vi "Termék megnyitás.vi"(8 "error in":errorcluster) -> (0 "error out":errorcluster, 2 "File name":string, 3 "Termék cluster array":T1[](array[typedef]))   [LabVIEW 2014]
panel:
  out "text":string
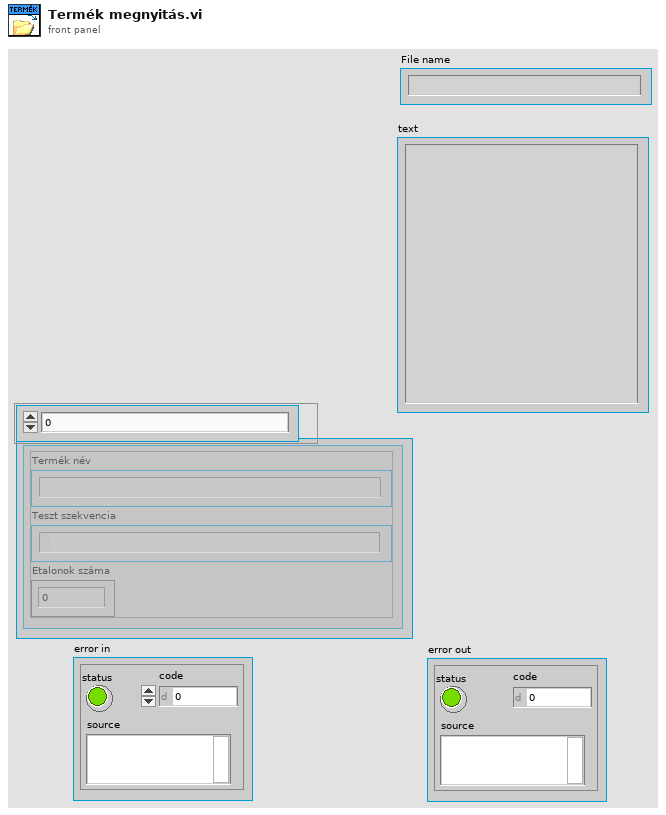
[diagram p1: front panel]
types:
  T1 = typedef "Termék cluster.ctl" = cluster{"Termék név":string, "Teszt szekvencia":path, "Etalonok száma":i8}
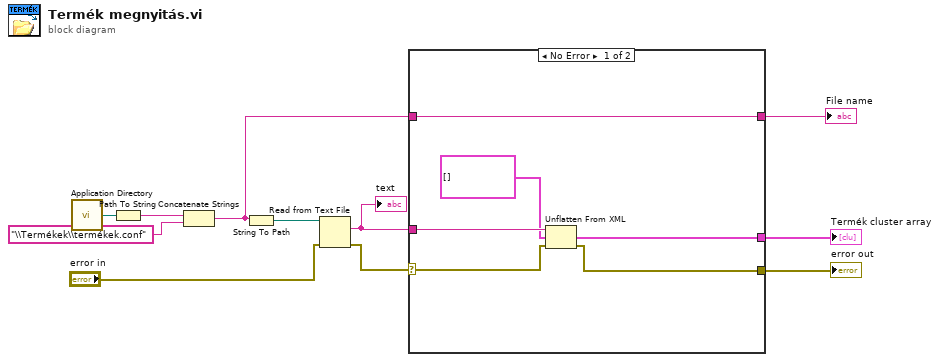
[diagram p0: block diagram]
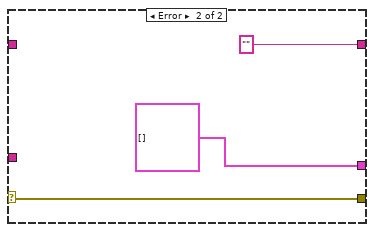
[diagram p2: hidden frame]
diagram:
  n1 = call <vilib>:"Application Directory.vi"() -> ("Application Directory"=w8:path)
  n2 = Path To String(path=w8) -> (string=w7:string)
  n3 = Concatenate Strings(w7, "\\Termékek\\termékek.conf" ("string")) -> (w2:string)
  n4 = String To Path(string=w2) -> (path=w5:path)
  n5 = Read from Text File(file (use dialog)=w5, error in="error in") -> (text=w11:string, error out=w10:errorcluster)  [unwired: 2 in, 2 out]
  "text" <- w11
  n6 = case shown="No Error" w10 {
    selector: w10 -> [w16 w20]
    tunnel: w11 -> [w17 _]
    tunnel: [w15 w20] -> w9
    tunnel: [w14 T1[] [] ("Termék cluster array")] -> w1
    tunnel: [w13 ""] -> w3
    tunnel: w2 -> [w13 _]
    frame No Error {
      n7 = Unflatten From XML(xml string=w17, type=T1[] [] ("Termék cluster array"), error in (no error)=w16) -> (value=w14:T1[], error out=w15:errorcluster)
    }
    frame Error {
    }
  }
  "error out" <- w9
  "File name" <- w3
  "Termék cluster array" <- w1
